vi "Weather FGV.vi"(7 "Weather FGV Method":T1, 8 "Error In":errorcluster, 10 "Query Interval (min)":dbl, 11 "Display Manager In":refnum<class "Display Manager.lvclass">) -> (0 "Error Out":errorcluster, 2 "Weather Data":T2, 3 "Display Manager Out":refnum<class "Display Manager.lvclass">)   [LabVIEW 2019, in "Display Manager.lvclass"]
uses:
  Display Manager.lvclass
  <vilib>/Memosfet/OpenWeatherAPI/Open Weather Session/Public/Controls/Weather Data.ctl
  <vilib>/Memosfet/OpenWeatherAPI/Open Weather Session/Public/Controls/Weather Sample Data.ctl
  <vilib>/Memosfet/OpenWeatherAPI/Open Weather Session/Public/Controls/Weather Description Data.ctl
  Controls/Weather FGV Method.ctl
  Accessors/Open Weather Session/Get Open Weather Session.vi
  <vilib>/Memosfet/OpenWeatherAPI/Open Weather Session/Open Weather Session.lvclass
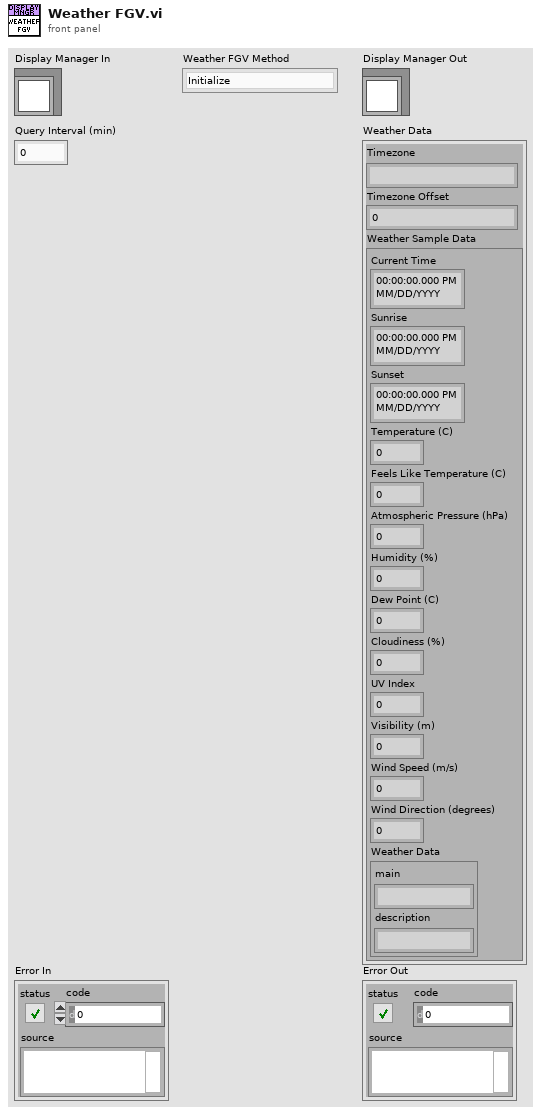
[diagram p1: front panel]
types:
  T1 = typedef "Display Manager.lvclass/Weather FGV Method.ctl" = enum16{"Initialize", "Query Weather"}
  T2 = typedef "Open Weather Session.lvclass/Weather Data.ctl" = cluster{"Timezone":string, "Timezone Offset":dbl, "Weather Sample Data":T3}
  T3 = typedef "Open Weather Session.lvclass/Weather Sample Data.ctl" = cluster{"Current Time":timestamp, "Sunrise":timestamp, "Sunset":timestamp, "Temperature (C)":dbl, "Feels Like Temperature (C)":dbl, "Atmospheric Pressure (hPa)":dbl, "Humidity (%)":dbl, "Dew Point (C)":dbl, "Cloudiness (%)":dbl, "UV Index":dbl, "Visibility (m)":dbl, "Wind Speed (m/s)":dbl, "Wind Direction (degrees)":dbl, "Weather Data":T4}
  T4 = typedef "Open Weather Session.lvclass/Weather Description Data.ctl" = cluster{"main":string, "description":string}
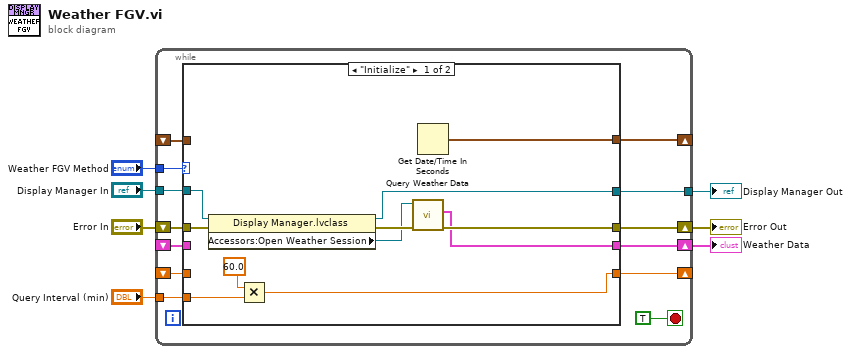
[diagram p0: block diagram]
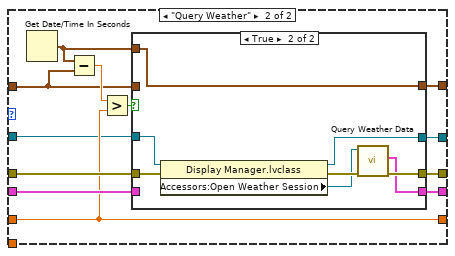
[diagram p2: hidden frame]
diagram:
  n1 = while {
    shift-right: [w20] -> w7
    shift-left: "Error In" -> [w18]
    shift-right: [w19] -> w6
    shift-left: _ -> [w16]
    tunnel: "Weather FGV Method" -> [w15]
    tunnel: "Query Interval (min)" -> [w10]
    shift-right: [w14] -> _
    shift-left: _ -> [w11]
    shift-right: [w13] -> _
    shift-left: _ -> [w12]
    tunnel: "Display Manager In" -> [w9]
    tunnel: [w8] -> w1
    stop <- TRUE stop-if-true
    n2 = case shown="\"Initialize\"" w15 {
      tunnel: [w30 w43] -> w20
      tunnel: [w29 w42] -> w19
      tunnel: w18 -> [w28 w41]
      tunnel: w16 -> [_ w40]
      tunnel: w11 -> [_ w38]
      tunnel: [w21 w38] -> w14
      tunnel: [w31 w35] -> w13
      tunnel: w12 -> [_ w34]
      tunnel: w10 -> [w23 _]
      tunnel: w9 -> [w25 w33]
      tunnel: [w24 w32] -> w8
      frame "Initialize" {
        n3 = property class="Display Manager.lvclass"(reference=w25, error in=w28) -> (reference out=w24:refnum<class "Display Manager.lvclass">, error out=w27:errorcluster, "Accessors:Open Weather Session"=w26:refnum<class "Open Weather Session.lvclass">)
        n4 = Multiply(x=60.0, y=w23) -> (x*y=w21:dbl)
        n5 = call-dynamic "Query Weather Data.vi"("Error In"=w27, "Open Weather Session In"=w26) -> ("Error Out"=w30:errorcluster, "Weather Data"=w29:T2)  [unwired: 7 in, 1 out]
        n6 = Get Date/Time In Seconds() -> (seconds since 1Jan1904=w31:timestamp)
      }
      frame "Query Weather" {
        n7 = Get Date/Time In Seconds() -> (seconds since 1Jan1904=w36:timestamp)
        n8 = Subtract(x=w36, y=w34) -> (x-y=w39:dbl)
        n9 = Greater?(x=w39, y=w38) -> (0:w37:bool)
        n10 = case shown="True" w37 {
          tunnel: [w46 w55] -> w43
          tunnel: [w47 w54] -> w42
          tunnel: w41 -> [w46 w52]
          tunnel: w40 -> [w47 _]
          tunnel: w36 -> [_ w53]
          tunnel: [w45 w53] -> w35
          tunnel: w34 -> [w45 _]
          tunnel: w33 -> [w44 w51]
          tunnel: [w44 w50] -> w32
          frame False {
          }
          frame True {
            n11 = property class="Display Manager.lvclass"(reference=w51, error in=w52) -> (reference out=w50:refnum<class "Display Manager.lvclass">, error out=w49:errorcluster, "Accessors:Open Weather Session"=w48:refnum<class "Open Weather Session.lvclass">)
            n12 = call-dynamic "Query Weather Data.vi"("Error In"=w49, "Open Weather Session In"=w48) -> ("Error Out"=w55:errorcluster, "Weather Data"=w54:T2)  [unwired: 7 in, 1 out]
          }
        }
      }
    }
  }
  "Error Out" <- w7
  "Weather Data" <- w6
  "Display Manager Out" <- w1
